vi "ULS Galvo.vi"(8 "error in (no error)":errorcluster, 10 "Galvo Degree":dbl format="%#_13g", 11 "IFD in":refnum<class "IFD.lvclass">) -> (0 "error out":errorcluster, 3 "IFD out":refnum<class "IFD.lvclass">)   [LabVIEW 2016, in "IFD.lvclass"]
uses:
  IFD.lvclass
  Tag/IFD_Tag.lvclass/IFD_Tag.ctl
  IFD.lvclass/IFD.ctl
  Tag/IFD_Tag.lvclass
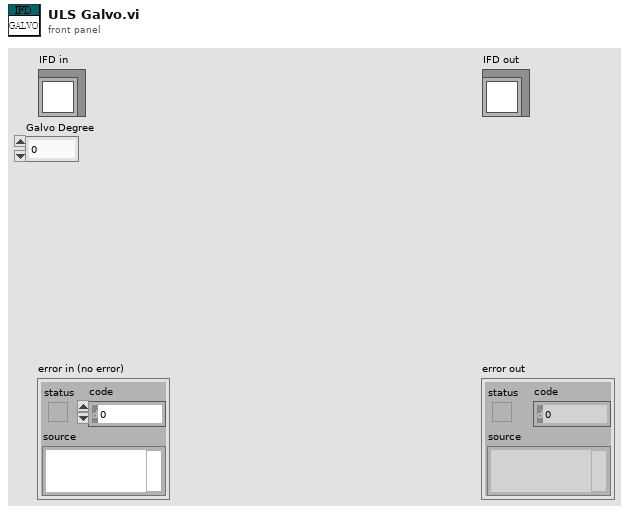
[diagram p1: front panel]
types:
  T1 = enum16{"Undefined(DO NOT USE)", "U8", "ASCII", "U16", "U32", "RATIONAL", "I8", "Undefined 8 bit", "I16", "I32", "SRATIONAL", "SGL", "DBL"}
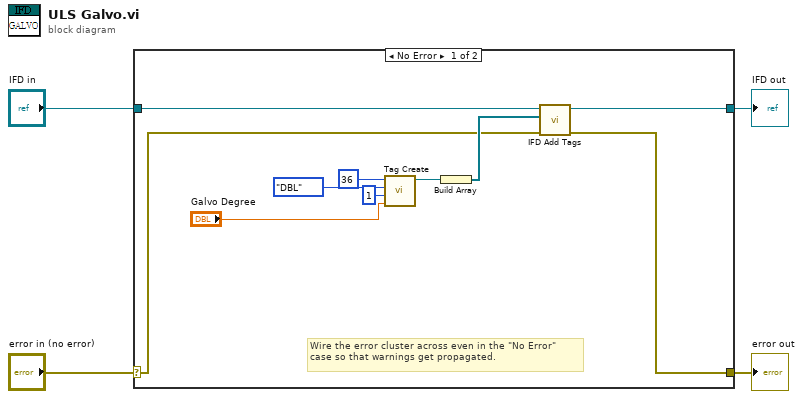
[diagram p0: block diagram]
diagram:
  n1 = case shown="No Error" "error in (no error)" {
    selector: "error in (no error)" -> [w6 w16]
    tunnel: [w5 w16] -> w3
    tunnel: [w13 w15] -> w1
    tunnel: "IFD in" -> [w14 w15]
    frame No Error {
      # "Wire the error cluster across even in the \"No Error\"\ncase so that warnings get propagated."
      n2 = call "Tag Create.vi"("Data"="Galvo Degree", "Data Count"=u32 1, "Data Type"=T1."DBL", "Tag ID"=u16 36) -> ("IFD_Tag out"=w10:refnum<class "IFD_Tag.lvclass">)  [unwired: 7 in]
      n3 = Build Array(w10) -> (w9:refnum<class "IFD_Tag.lvclass">[])
      n4 = call "IFD Add Tags.vi"("error in (no error)"=w6, "Tag(s)"=w9, "IFD in"=w14) -> ("error out"=w5:errorcluster, "IFD out"=w13:refnum<class "IFD.lvclass">)  [unwired: 7 in]
    }
    frame Error {
    }
  }
  "error out" <- w3
  "IFD out" <- w1
